vi "ReadWrite Config.vi"(6 "Write":bool, 8 "Error In":errorcluster, 10 "IoT Parameters":T1={"MQTT Broker"={"address (IP)"="azwqv45vu9vjz.iot.us-east-2.amazonaws.com", "port"=8883}, "cert path"={"client cert file"=path "C:/Users/Jembedded/Downloads/aa6df4a004-certificate.pem.crt", "client key file"=path "C:/Users/Jembedded/Downloads/aa6df4a004-private.pem.key"}, "Topic Prefix"="", "Serial Number"="", "Subscriptions"=[]}, 11 "Path":path) -> (0 "Error Out":errorcluster, 2 "IoT Parameters out":T1={"MQTT Broker"={"address (IP)"="azwqv45vu9vjz.iot.us-east-2.amazonaws.com", "port"=8883}, "cert path"={"client cert file"=path "C:/Users/Jembedded/Downloads/aa6df4a004-certificate.pem.crt", "client key file"=path "C:/Users/Jembedded/Downloads/aa6df4a004-private.pem.key"}, "Topic Prefix"="", "Serial Number"="", "Subscriptions"=[]})   [LabVIEW 2018]
uses:
  Controls/IoT Parameters.ctl
  Controls/certs.ctl
  AWS_IoT.lvlib
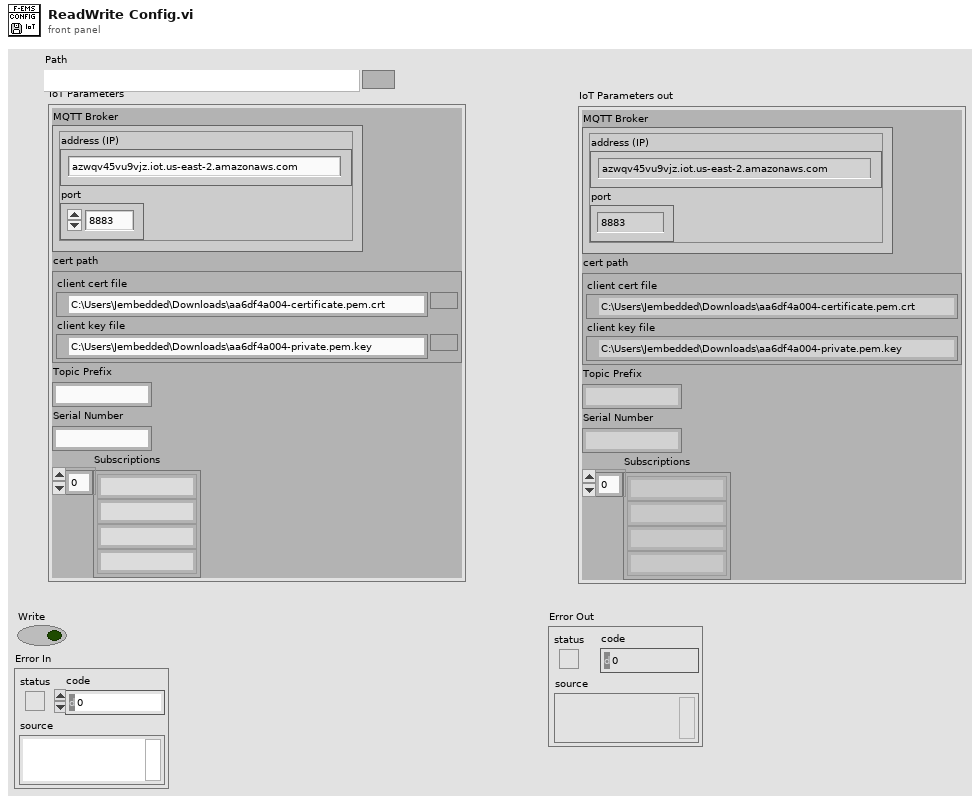
[diagram p1: front panel]
types:
  T1 = typedef "IoT Parameters.ctl" = cluster{"MQTT Broker":cluster{"address (IP)":string, "port":u16}, "cert path":T2, "Topic Prefix":string, "Serial Number":string, "Subscriptions":string[]}
  T2 = typedef "AWS_IoT.lvlib/certs.ctl" = cluster{"client cert file":path, "client key file":path}
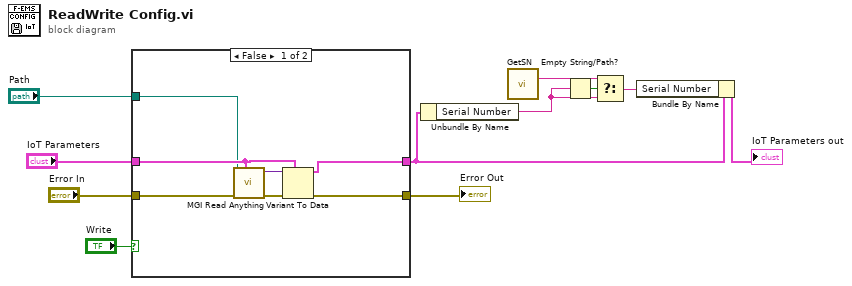
[diagram p0: block diagram]
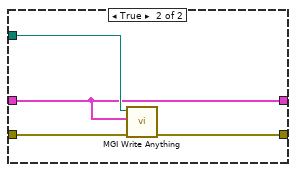
[diagram p2: hidden frame]
diagram:
  n1 = case shown="False" "Write" {
    tunnel: [w15 w22] -> w10
    tunnel: "Error In" -> [w16 w21]
    tunnel: "IoT Parameters" -> [w14 w19]
    tunnel: "Path" -> [w12 w20]
    tunnel: [w13 w19] -> w6
    frame False {
      n2 = call <userlib>:"MGI Read Anything.vi"("Type of Anything"=w14, "Error In"=w16, "Path (dialog)"=w12) -> ("Error Out"=w18:errorcluster, "Anything"=w17:variant)  [unwired: 5 in, 2 out]
      n3 = Variant To Data(error in=w18, type=w14, Variant=w17) -> (data=w13:T1, error out=w15:errorcluster)
    }
    frame True {
      n4 = call <userlib>:"MGI Write Anything.vi"("Error In"=w21, "Anything"=w19, "Path (dialog)"=w20) -> ("Error Out"=w22:errorcluster)  [unwired: 6 in, 2 out]
    }
  }
  "Error Out" <- w10
  n5 = Unbundle By Name(w6) -> ("Serial Number"=w3:string)
  n6 = call "GetSN.vi"() -> ("SN"=w4:string)  [unwired: 10 in, 1 out]
  n7 = Empty String/Path?(string/path=w3) -> (empty?=w5:bool)
  n8 = Select(t=w4, s=w5, f=w3) -> (s? t:f=w1:string)
  n9 = Bundle By Name(cluster=w6, "Serial Number"=w1) -> (→"IoT Parameters out":T1)
